vi "Method.vi"(4 "Value":refnum<class "Abs_Double Float.lvclass">) -> (1 "Result":refnum<class "Abs_Double Float.lvclass">)   [LabVIEW 2021, in "Increment_CPLX_DBL.lvclass"]
uses:
  Increment_CPLX_DBL.lvclass
  Abs_Types/Double Float/Abs_Double Float.lvclass
  C:/TSA/LV_Abstract/Source/Functions/Support/Function/One Terminal/DBL/AbsFunc_One Term_DBL.lvclass
  C:/Program Files (x86)/National Instruments/LabVIEW 2021/vi.lib/TSA/Abstract Data Classes/Abs_Types/Double Float/Abs_Double Float.lvclass
  Support/Function/One Terminal/DBL/AbsFunc_One Term_DBL.lvclass/AbsFunc_One Term_DBL.ctl
  Support/Function/One Terminal/DBL/Properties/Write Numeric A.vi
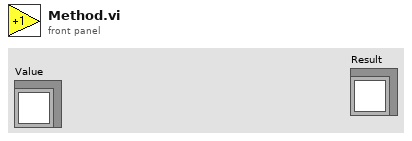
[diagram p1: front panel]
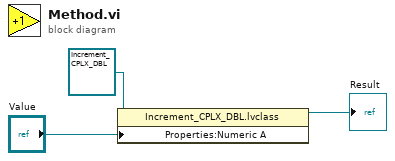
[diagram p0: block diagram]
diagram:
  n1 = property class="Increment_CPLX_DBL.lvclass"(reference=refnum<class "Increment_CPLX_DBL.lvclass"> refnum ("Decrement_DBL.lvclass"), "Properties:Numeric A"="Value") -> (reference out=→"Result":refnum<class "Increment_CPLX_DBL.lvclass">)  [unwired: 1 in, 1 out]
